vi "No Fire Test.vi"(8 "error in (no error)":errorcluster, 10 "Switch Resource Name":refnum<visa-resource-name>="COM12", 11 "Keithley Resource Name":refnum<visa-resource-name>="COM12") -> (0 "error out":errorcluster, 1 "No-Fire Results BW2":T1={"Current"=["7.203409E-06\n", "7.484487E-06\n", "7.484465E-06\n", "8.327806E-06\n", "7.765564E-06\n", "7.062867E-06\n", "8.187235E-06\n", "8.187257E-06\n", "7.906143E-06\n", "7.765622E-06\n", "7.203482E-06\n", "7.484487E-06\n", "7.484487E-06\n", "7.625029E-06\n", "7.765600E-06\n", "7.203387E-06\n", "7.625014E-06\n", "7.765651E-06\n", "8.046671E-06\n", "7.906223E-06\n", "7.343981E-06\n", "7.203409E-06\n", "7.625109E-06\n", "7.765608E-06\n", "7.906143E-06\n", "8.187286E-06\n", "8.046729E-06\n", "7.484501E-06\n", "8.046707E-06\n", "7.906157E-06\n", "7.484501E-06\n", "7.062881E-06\n", "7.906165E-06\n", "7.625087E-06\n", "7.906179E-06\n", "7.765622E-06\n", "7.765593E-06\n", "7.343951E-06\n", "7.906230E-06\n", "7.625087E-06\n", "7.062867E-06\n", "7.484530E-06\n", "7.906172E-06\n", "7.906157E-06\n", "7.625029E-06\n", "7.906143E-06\n", "7.625073E-06\n", "7.343959E-06\n", "8.187249E-06\n", "8.187220E-06\n", "8.187286E-06\n", "7.906172E-06\n", "7.484487E-06\n", "7.765608E-06\n", "7.625073E-06\n", "7.906172E-06\n", "7.906179E-06\n", "7.484523E-06\n", "7.625051E-06\n", "7.765593E-06\n", "7.484559E-06\n", "7.765637E-06\n", "7.484581E-06\n", "8.046714E-06\n", "7.765630E-06\n", "7.765651E-06\n", "8.187286E-06\n", "8.046707E-06\n", "7.906143E-06\n", "8.046729E-06\n", "7.906143E-06\n", "8.046773E-06\n", "7.625065E-06\n", "7.344046E-06\n", "8.327836E-06\n", "7.765644E-06\n", "7.765630E-06\n", "7.484545E-06\n", "7.765615E-06\n", "7.765644E-06\n", "7.203424E-06\n", "7.906143E-06\n", "7.484523E-06\n", "8.046758E-06\n", "7.765666E-06\n", "7.906165E-06\n", "7.625073E-06\n", "8.327777E-06\n", "7.484523E-06\n", "7.625073E-06\n", "7.906150E-06\n", "7.625065E-06\n", "7.625065E-06\n", "7.765630E-06\n", "7.625124E-06\n", "7.765615E-06\n", "7.484494E-06\n", "7.343966E-06\n", "7.906216E-06\n", "7.765608E-06\n", "7.906194E-06\n", "7.484581E-06\n", "7.765622E-06\n", "7.906208E-06\n", "7.343973E-06\n", "7.062918E-06\n", "7.343981E-06\n", "7.765579E-06\n", "7.484530E-06\n", "7.765637E-06\n", "7.625087E-06\n", "8.046707E-06\n", "8.468349E-06\n", "7.906179E-06\n", "7.625065E-06\n", "7.906150E-06\n", "7.906194E-06\n", "7.765644E-06\n", "7.765622E-06\n", "8.187257E-06\n", "7.484501E-06\n", "7.765608E-06\n", "7.343973E-06\n", "7.906143E-06\n", "7.625051E-06\n", "7.906150E-06\n", "7.765593E-06\n", "7.625044E-06\n", "7.765622E-06\n", "7.625102E-06\n", "7.343959E-06\n", "7.484588E-06\n", "7.765622E-06\n", "7.625109E-06\n", "7.906172E-06\n", "7.343973E-06\n", "7.625102E-06\n", "8.468385E-06\n", "7.906201E-06\n", "7.906194E-06\n", "8.046707E-06\n", "7.625109E-06\n", "7.906172E-06\n", "7.906179E-06\n", "8.046773E-06\n", "7.906216E-06\n", "8.327799E-06\n", "7.906223E-06\n", "7.343995E-06\n", "8.046714E-06\n", "8.046685E-06\n"], "Voltage"=[], "Time"=[]}, 2 "No-Fire Results BW1":T1={"Current"=["7.203409E-06\n", "7.484487E-06\n", "7.484465E-06\n", "8.327806E-06\n", "7.765564E-06\n", "7.062867E-06\n", "8.187235E-06\n", "8.187257E-06\n", "7.906143E-06\n", "7.765622E-06\n", "7.203482E-06\n", "7.484487E-06\n", "7.484487E-06\n", "7.625029E-06\n", "7.765600E-06\n", "7.203387E-06\n", "7.625014E-06\n", "7.765651E-06\n", "8.046671E-06\n", "7.906223E-06\n", "7.343981E-06\n", "7.203409E-06\n", "7.625109E-06\n", "7.765608E-06\n", "7.906143E-06\n", "8.187286E-06\n", "8.046729E-06\n", "7.484501E-06\n", "8.046707E-06\n", "7.906157E-06\n", "7.484501E-06\n", "7.062881E-06\n", "7.906165E-06\n", "7.625087E-06\n", "7.906179E-06\n", "7.765622E-06\n", "7.765593E-06\n", "7.343951E-06\n", "7.906230E-06\n", "7.625087E-06\n", "7.062867E-06\n", "7.484530E-06\n", "7.906172E-06\n", "7.906157E-06\n", "7.625029E-06\n", "7.906143E-06\n", "7.625073E-06\n", "7.343959E-06\n", "8.187249E-06\n", "8.187220E-06\n", "8.187286E-06\n", "7.906172E-06\n", "7.484487E-06\n", "7.765608E-06\n", "7.625073E-06\n", "7.906172E-06\n", "7.906179E-06\n", "7.484523E-06\n", "7.625051E-06\n", "7.765593E-06\n", "7.484559E-06\n", "7.765637E-06\n", "7.484581E-06\n", "8.046714E-06\n", "7.765630E-06\n", "7.765651E-06\n", "8.187286E-06\n", "8.046707E-06\n", "7.906143E-06\n", "8.046729E-06\n", "7.906143E-06\n", "8.046773E-06\n", "7.625065E-06\n", "7.344046E-06\n", "8.327836E-06\n", "7.765644E-06\n", "7.765630E-06\n", "7.484545E-06\n", "7.765615E-06\n", "7.765644E-06\n", "7.203424E-06\n", "7.906143E-06\n", "7.484523E-06\n", "8.046758E-06\n", "7.765666E-06\n", "7.906165E-06\n", "7.625073E-06\n", "8.327777E-06\n", "7.484523E-06\n", "7.625073E-06\n", "7.906150E-06\n", "7.625065E-06\n", "7.625065E-06\n", "7.765630E-06\n", "7.625124E-06\n", "7.765615E-06\n", "7.484494E-06\n", "7.343966E-06\n", "7.906216E-06\n", "7.765608E-06\n", "7.906194E-06\n", "7.484581E-06\n", "7.765622E-06\n", "7.906208E-06\n", "7.343973E-06\n", "7.062918E-06\n", "7.343981E-06\n", "7.765579E-06\n", "7.484530E-06\n", "7.765637E-06\n", "7.625087E-06\n", "8.046707E-06\n", "8.468349E-06\n", "7.906179E-06\n", "7.625065E-06\n", "7.906150E-06\n", "7.906194E-06\n", "7.765644E-06\n", "7.765622E-06\n", "8.187257E-06\n", "7.484501E-06\n", "7.765608E-06\n", "7.343973E-06\n", "7.906143E-06\n", "7.625051E-06\n", "7.906150E-06\n", "7.765593E-06\n", "7.625044E-06\n", "7.765622E-06\n", "7.625102E-06\n", "7.343959E-06\n", "7.484588E-06\n", "7.765622E-06\n", "7.625109E-06\n", "7.906172E-06\n", "7.343973E-06\n", "7.625102E-06\n", "8.468385E-06\n", "7.906201E-06\n", "7.906194E-06\n", "8.046707E-06\n", "7.625109E-06\n", "7.906172E-06\n", "7.906179E-06\n", "8.046773E-06\n", "7.906216E-06\n", "8.327799E-06\n", "7.906223E-06\n", "7.343995E-06\n", "8.046714E-06\n", "8.046685E-06\n"], "Voltage"=[], "Time"=[]}, 3 "Test Status":string, 5 "Stop Status":bool)   [LabVIEW 2018]
uses:
  Custom Controls/No Fire State.ctl
  Door Status Global Variable.vi
  Agilent 34970/Agilent 34970.lvlib
panel:
  in  "No Fire State":T2
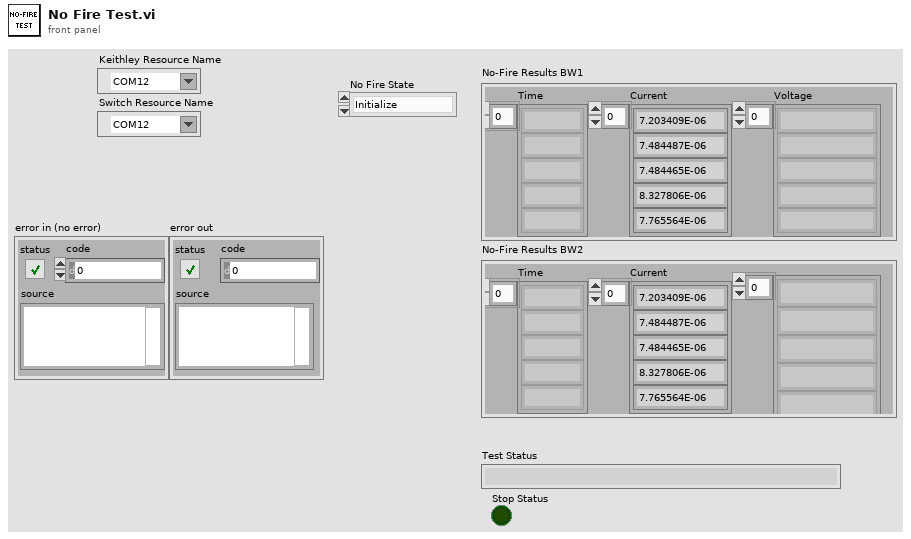
[diagram p1: front panel]
types:
  T1 = cluster{"Current":string[], "Voltage":string[], "Time":string[]}
  T2 = typedef "No Fire State.ctl" = enum16{"Initialize", "Switch BW 1", "No Fire BW 1", "Switch BW 2", "No Fire BW 2", "Stop"}
  T3 = enum16{"None", "XON / XOFF", "RTS / CTS", "DTR / DSR"}
  T4 = enum16{"1200", "2400", "4800", "9600", "19200", "38400", "57600", "115200"}
  T5 = cluster{"Timeout Value (10000)":u32, "Baud Rate (57600)":enum16{"1200", "2400", "4800", "9600", "19200", "38400", "57600", "115200"}, "Flow Control (1:XON/XOFF)":enum16{"None", "XON / XOFF", "RTS / CTS", "DTR / DSR"}}
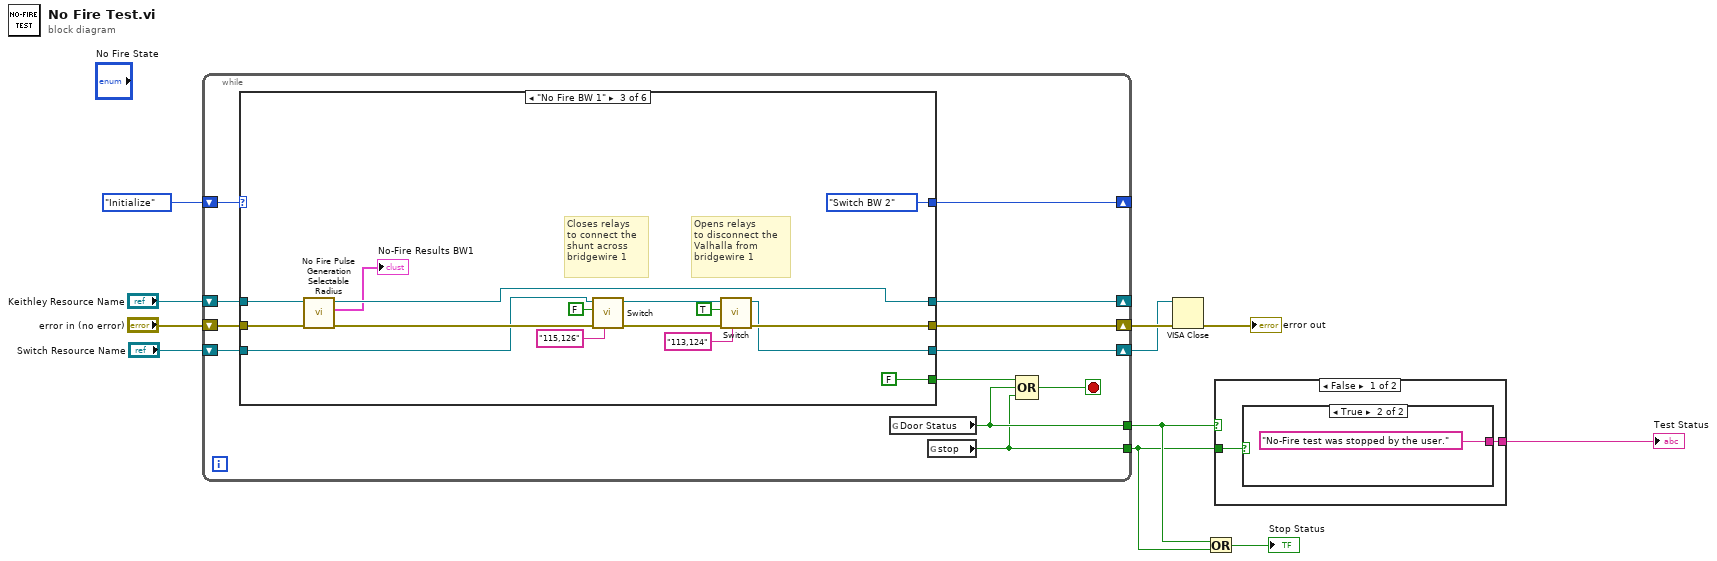
[diagram p0: block diagram]
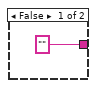
[diagram p2: hidden frame]
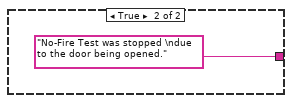
[diagram p3: hidden frame]
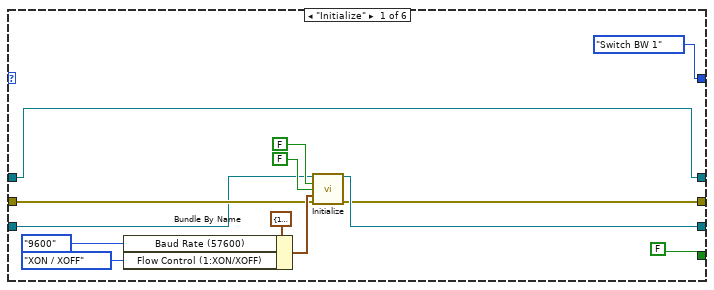
[diagram p4: hidden frame]
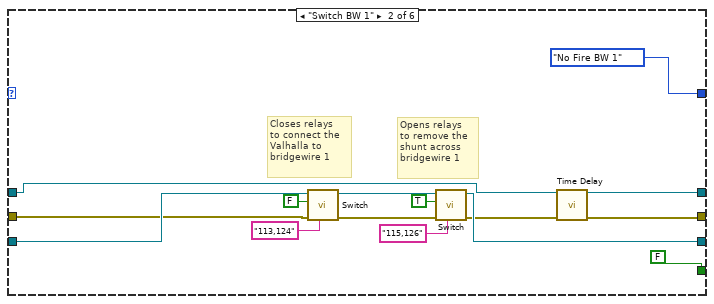
[diagram p5: hidden frame]
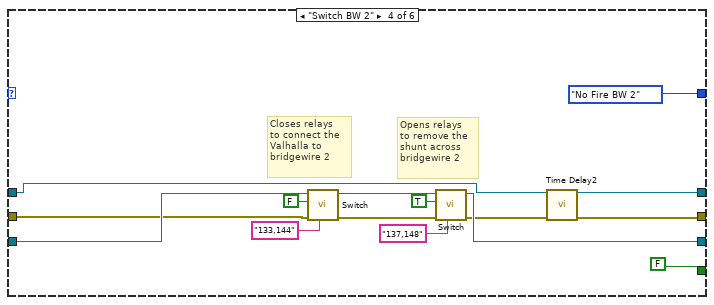
[diagram p6: hidden frame]
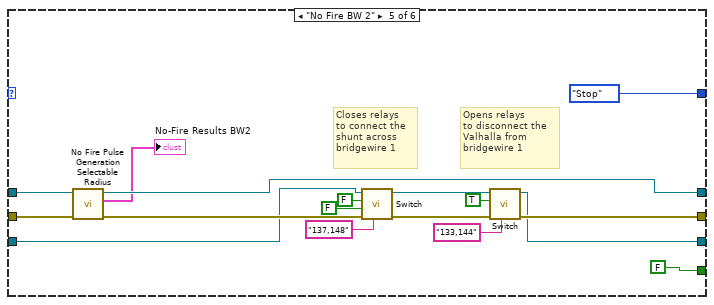
[diagram p7: hidden frame]
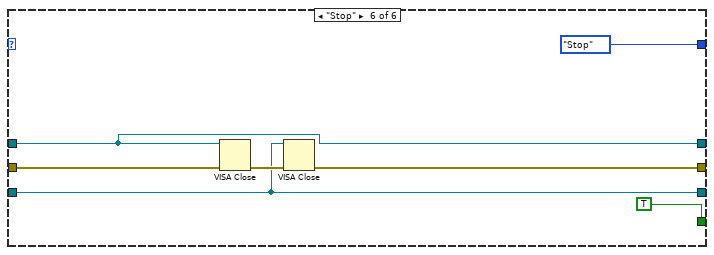
[diagram p8: hidden frame]
diagram:
  n1 = while {
    shift-right: [w22] -> w7
    shift-left: "error in (no error)" -> [w23]
    shift-right: [w20] -> _
    shift-left: "Keithley Resource Name" -> [w21]
    shift-right: [w17] -> _
    shift-left: No_Fire_State."Initialize" ("No Fire State") -> [w19]
    shift-right: [w16] -> w5
    shift-left: "Switch Resource Name" -> [w18]
    tunnel: [w13] -> w3
    tunnel: [w12] -> w1
    stop <- w14 stop-if-true
    n2 = case shown="\"No Fire BW 1\"" w19 {
      tunnel: [No_Fire_State."Switch BW 1" ("No Fire State") No_Fire_State."No Fire BW 1" ("No Fire State") No_Fire_State."Switch BW 2" ("No Fire State") No_Fire_State."No Fire BW 2" ("No Fire State") No_Fire_State."Stop" ("No Fire State") No_Fire_State."Stop" ("No Fire State")] -> w17
      tunnel: w23 -> [w30 w43 w65 w73 w96 w102]
      tunnel: [w26 w38 w61 w68 w92 w101] -> w22
      tunnel: w21 -> [w25 w41 w64 w71 w95 w99]
      tunnel: [w25 w41 w62 w71 w93 w99] -> w20
      tunnel: w18 -> [w27 w49 w60 w79 w91 w100]
      tunnel: [w29 w42 w59 w72 w90 w100] -> w16
      tunnel: [FALSE FALSE FALSE FALSE FALSE TRUE] -> w15
      frame "Initialize" {
        n3 = Bundle By Name(cluster=T5 {"Timeout Value (10000)"=10000, "Baud Rate (57600)"=enum."9600", "Flow Control (1:XON/XOFF)"=enum."XON / XOFF"} ("Serial Port Configuration"), "Baud Rate (57600)"=T4."9600", "Flow Control (1:XON/XOFF)"=T3."XON / XOFF") -> (w34:T5)
        n4 = call "Initialize.vi"("VISA Resource Name"=w27, "ID Query (T: Check)"=FALSE, "Reset (T: Reset)"=FALSE, "Serial Port Configuration"=w34, "error in (no error)"=w30) -> ("VISA Resource Name Out"=w29:refnum<visa-resource-name>, "error out"=w26:errorcluster)  [unwired: 9 in]
      }
      frame "Switch BW 1" {
        # "Opens relays\nto remove the \nshunt across \nbridgewire 1"
        # "Closes relays\nto connect the \nValhalla to \nbridgewire 1"
        n5 = call "Switch.vi"("Channel List(empty)"="113,124", "error in (no error)"=w43, "Open/Close (F:Close)"=FALSE, "VISA Resource Name"=w49) -> ("error out"=w44:errorcluster, "VISA Resource Name Out"=w46:refnum<visa-resource-name>)  [unwired: 5 in, 1 out]
        n6 = call "Switch.vi"("Channel List(empty)"="115,126", "error in (no error)"=w44, "Open/Close (F:Close)"=TRUE, "VISA Resource Name"=w46) -> ("error out"=w39:errorcluster, "VISA Resource Name Out"=w42:refnum<visa-resource-name>)  [unwired: 5 in, 1 out]
        n7 = call "Time Delay"("error in (no error)"=w39) -> ("error out"=w38:errorcluster)  [unwired: 10 in]
      }
      frame "No Fire BW 1" {
        # "Closes relays\nto connect the \nshunt across \nbridgewire 1"
        # "Opens relays\nto disconnect the \nValhalla from \nbridgewire 1"
        n8 = call "No Fire Pulse Generation Selectable Radius.vi"("error in (no error)"=w65, "VISA resource name"=w64) -> ("error out"=w63:errorcluster, "No-Fire Results"=→"No-Fire Results BW1":T1, "VISA resource name out"=w62:refnum<visa-resource-name>)  [unwired: 7 in]
        n9 = call "Switch.vi"("Channel List(empty)"="115,126", "error in (no error)"=w63, "Open/Close (F:Close)"=FALSE, "VISA Resource Name"=w60) -> ("error out"=w57:errorcluster, "VISA Resource Name Out"=w56:refnum<visa-resource-name>)  [unwired: 5 in, 1 out]
        n10 = call "Switch.vi"("Channel List(empty)"="113,124", "error in (no error)"=w57, "Open/Close (F:Close)"=TRUE, "VISA Resource Name"=w56) -> ("error out"=w61:errorcluster, "VISA Resource Name Out"=w59:refnum<visa-resource-name>)  [unwired: 5 in, 1 out]
      }
      frame "Switch BW 2" {
        # "Opens relays\nto remove the \nshunt across \nbridgewire 2"
        # "Closes relays\nto connect the \nValhalla to \nbridgewire 2"
        n11 = call "Switch.vi"("Channel List(empty)"="133,144", "error in (no error)"=w73, "Open/Close (F:Close)"=FALSE, "VISA Resource Name"=w79) -> ("error out"=w74:errorcluster, "VISA Resource Name Out"=w76:refnum<visa-resource-name>)  [unwired: 5 in, 1 out]
        n12 = call "Switch.vi"("Channel List(empty)"="137,148", "error in (no error)"=w74, "Open/Close (F:Close)"=TRUE, "VISA Resource Name"=w76) -> ("error out"=w69:errorcluster, "VISA Resource Name Out"=w72:refnum<visa-resource-name>)  [unwired: 5 in, 1 out]
        n13 = call "Time Delay2"("error in (no error)"=w69) -> ("error out"=w68:errorcluster)  [unwired: 10 in]
      }
      frame "No Fire BW 2" {
        # "Closes relays\nto connect the \nshunt across \nbridgewire 1"
        # "Opens relays\nto disconnect the \nValhalla from \nbridgewire 1"
        n14 = call "No Fire Pulse Generation Selectable Radius.vi"("error in (no error)"=w96, "VISA resource name"=w95) -> ("error out"=w94:errorcluster, "No-Fire Results"=→"No-Fire Results BW2":T1, "VISA resource name out"=w93:refnum<visa-resource-name>)  [unwired: 7 in]
        n15 = call "Switch.vi"("Channel List(empty)"="137,148", "error in (no error)"=w94, "Close Exclusive (F:Normal)"=FALSE, "Open/Close (F:Close)"=FALSE, "VISA Resource Name"=w91) -> ("error out"=w88:errorcluster, "VISA Resource Name Out"=w87:refnum<visa-resource-name>)  [unwired: 4 in, 1 out]
        n16 = call "Switch.vi"("Channel List(empty)"="133,144", "error in (no error)"=w88, "Open/Close (F:Close)"=TRUE, "VISA Resource Name"=w87) -> ("error out"=w92:errorcluster, "VISA Resource Name Out"=w90:refnum<visa-resource-name>)  [unwired: 5 in, 1 out]
      }
      frame "Stop" {
        n17 = VISA Close(VISA resource name=w99, error in (no error)=w102) -> (error out=w103:errorcluster)
        n18 = VISA Close(VISA resource name=w100, error in (no error)=w103) -> (error out=w101:errorcluster)
      }
    }
    n19 = global read "Door Status Global Variable.vi" "Door Status"() -> (w13:bool)
    n20 = global read "Door Status Global Variable.vi" "stop"() -> (w12:bool)
    n21 = Compound Arithmetic op=OR(w15, w13, w12) -> (w14:bool)
  }
  n22 = VISA Close(VISA resource name=w5, error in (no error)=w7) -> (error out=→"error out":errorcluster)
  n23 = Or(x=w3, y=w1) -> (x .or. y?=→"Stop Status":bool)
  n24 = case shown="False" w3 {
    tunnel: [w105 "No-Fire Test was stopped \ndue to the door being opened." ("Test Status")] -> w2
    tunnel: w1 -> [w106 _]
    frame False {
      n25 = case shown="True" w106 {
        tunnel: ["" ("Test Status") "No-Fire test was stopped by the user." ("Test Status")] -> w105
        frame False {
        }
        frame True {
        }
      }
    }
    frame True {
    }
  }
  "Test Status" <- w2
